vi "DB Get Stations.vi"(8 "error in (no error)":errorcluster, 10 "Station Type":string) -> (0 "error out":errorcluster, 2 "Stations":string[](array[string]))   [LabVIEW 2019, in "Control Experiment.lvclass"]
uses:
  Control Experiment.lvclass
  <userlib>/LevyLab/LV-Data/LV-Data.PG/LV-Data.PGSQL.lvclass
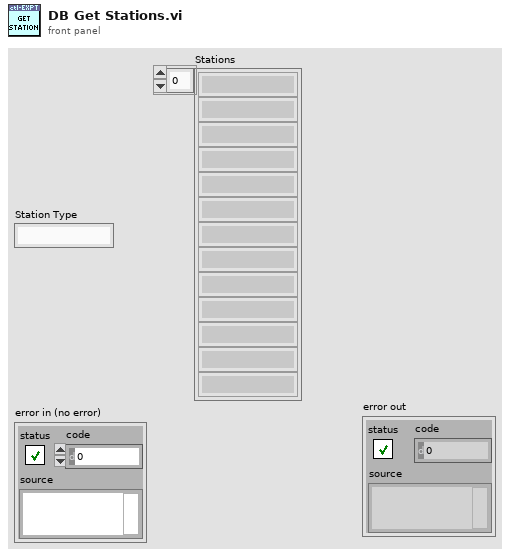
[diagram p1: front panel]
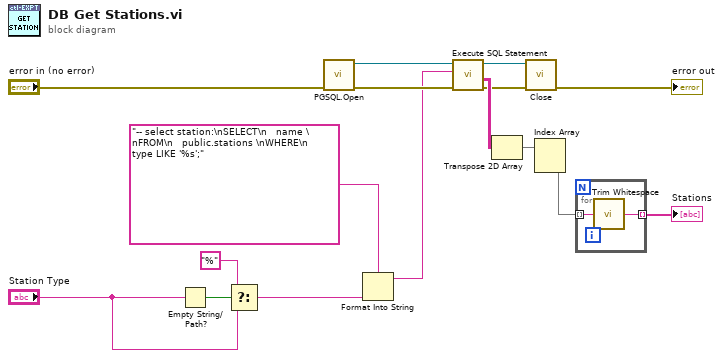
[diagram p0: block diagram]
diagram:
  n1 = Empty String/Path?(string/path="Station Type") -> (empty?=w14:bool)
  n2 = Select(t="%", s=w14, f="Station Type") -> (s? t:f=w13:string)
  n3 = call <userlib>:"PGSQL.Open.vi"("error in (no error)"="error in (no error)") -> ("error out"=w7:errorcluster, "Data.PG out"=w10:refnum<class "LV-Data.PGSQL.lvclass">)  [unwired: 9 in]
  n4 = Format Into String(format string="-- select station:\nSELECT\n   name \nFROM\n   public.stations \nWHERE\n   type LIKE '%s';" ("Address"), w13) -> (resulting string=w4:string)  [unwired: 2 in, 1 out]
  n5 = call <userlib>:"Execute SQL Statement.vi"("error in (no error)"=w7, "SQL string"=w4, "Data.PGQL in"=w10) -> ("error out"=w6:errorcluster, "Result"=w8:string[][], "Data.PGSQL out"=w9:refnum<class "LV-Data.PGSQL.lvclass">)  [unwired: 6 in]
  n6 = Transpose 2D Array(2D array=w8) -> (transposed array=w5:string[][])
  n7 = call-dynamic "Close.vi"("error in (no error)"=w6, "Data.PG in"=w9) -> ("error out"=→"error out":errorcluster)  [unwired: 8 in, 1 out]
  n8 = Index Array(array=w5) -> (element=w2:string[])  [unwired: 2 in]
  n9 = for {
    tunnel: w2 -> [w18] mode=indexing
    tunnel: [w17] -> w16 mode=indexing
    n10 = call <vilib>:"Trim Whitespace.vi"("string"=w18) -> ("trimmed string"=w17:string)  [unwired: 1 in]
  }
  "Stations" <- w16
